vi "Force Move LogFiles.vi"(8 "error in":errorcluster, 10 "Force Move":bool, 11 "KIT-QVA in":refnum<class "KIT-QVA.lvclass">) -> (0 "error out":errorcluster, 3 "KIT-QVA out":refnum<class "KIT-QVA.lvclass">)   [LabVIEW 2016, in "KIT-QVA.lvlib" / "KIT-QVA.lvclass"]
doc: "Public interface to force move quench log-files."
uses:
  KIT-QVA.lvclass
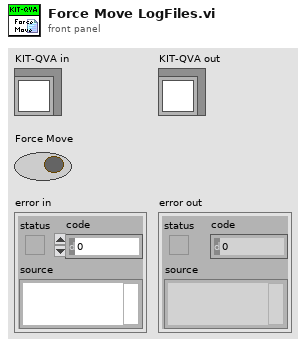
[diagram p1: front panel]
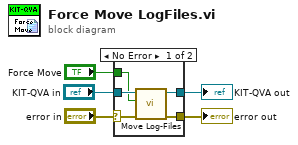
[diagram p0: block diagram]
diagram:
  n1 = case shown="No Error" "error in" {
    selector: "error in" -> [w8 w12]
    tunnel: [w7 w12] -> w4
    tunnel: [w9 w11] -> w2
    tunnel: "KIT-QVA in" -> [w10 w11]
    tunnel: "Force Move" -> [w6 _]
    frame No Error {
      n2 = call "Move Log-Files.vi"("error in"=w8, "Force Move"=w6, "KIT-QVA in"=w10) -> ("error out"=w7:errorcluster, "KIT-QVA out"=w9:refnum<class "KIT-QVA.lvclass">)  [unwired: 7 in]
    }
    frame Error {
    }
  }
  "error out" <- w4
  "KIT-QVA out" <- w2
